vi "SizeFromTau.vi"(7 "Variables":T1={"Boltzmans "=1.3806e-23, "Temp K"=293.0, "Viscosity"=0.00089, "lamda (m)"=6.4e-07, "n"=1.33}, 10 "Angle (degrees)":dbl=90.0, 11 "tau 1/s":dbl) -> (1 "damping (ms)":dbl, 2 "size (um)":dbl)   [LabVIEW 2022 SP3]
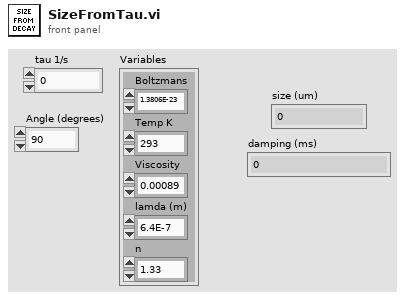
[diagram p1: front panel]
types:
  T1 = cluster{"Boltzmans ":dbl, "Temp K":dbl, "Viscosity":dbl, "lamda (m)":dbl, "n":dbl}
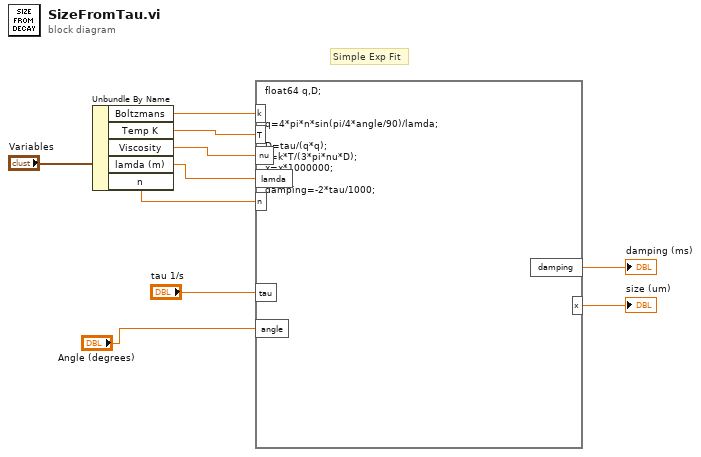
[diagram p0: block diagram]
diagram:
  # "Simple Exp Fit"
  n1 = Unbundle By Name("Variables") -> ("Boltzmans"=w10:dbl, "Temp K"=w9:dbl, "Viscosity"=w8:dbl, "lamda (m)"=w7:dbl, "n"=w6:dbl)
  n2 = formula code="float64 q,D;\n\n\nq=4*pi*n*sin(pi/4*angle/90)/lamda;\n\nD=tau/(q*q);\nx=k*T/(3*pi*nu*D);\nx=x*1000000;\n\ndamping=-2*tau/1000;"("k"=w10, "T"=w9, "nu"=w8, "lamda"=w7, "n"=w6, "tau"="tau 1/s", "angle"="Angle (degrees)") -> ("x"=→"size (um)":dbl, "damping"=→"damping (ms)":dbl)
